vi "main.vi"() -> ()   [LabVIEW 2025]
uses:
  <vilib>/Utility/file.llb/Write Delimited Spreadsheet (DBL).vi
panel:
  out "output array":dbl[][](array[numeric])
  in  "Scrivi su File":bool
  out "Outlet":dbl
  out "Secondary":dbl
  out "Primary":dbl
  out "Waveform Graph":dynamicdata(graph)
  in  "Stop Button":bool
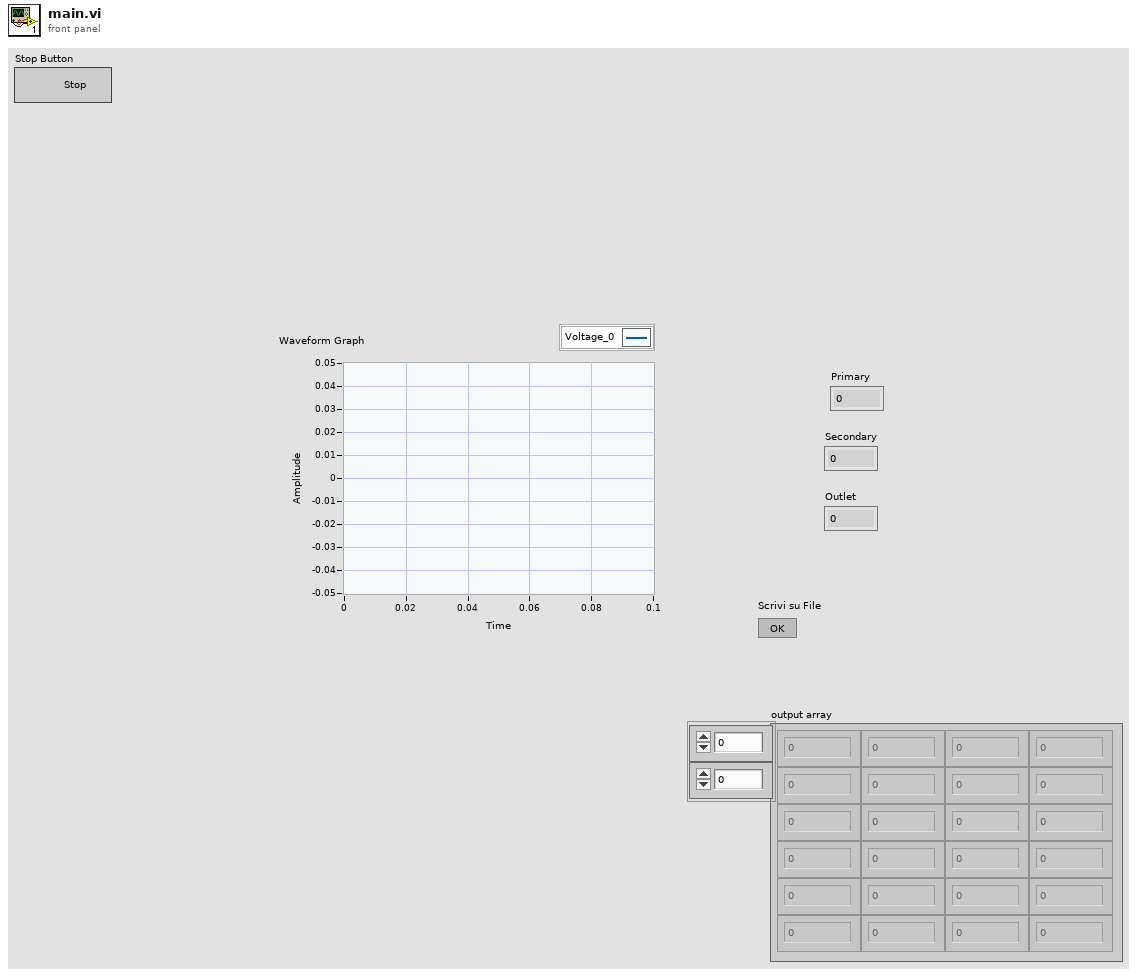
[diagram p1: front panel]
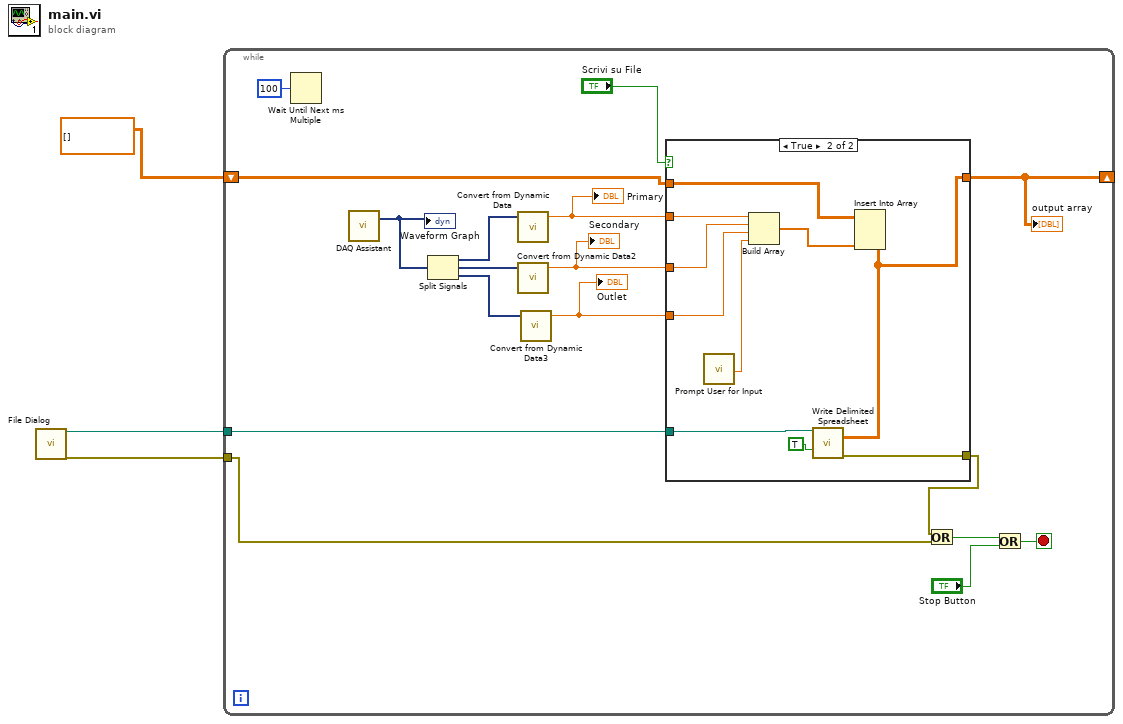
[diagram p0: block diagram]
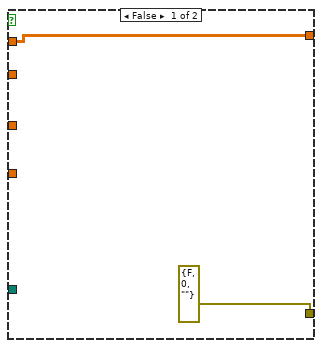
[diagram p2: hidden frame]
diagram:
  n1 = call "File Dialog"() -> ("selected path"=w3:path, "error out"=w2:errorcluster)  [unwired: 12 in, 2 out]
  n2 = while {
    tunnel: w3 -> [w9]
    tunnel: w2 -> [w7]
    shift-right: [w4] -> _
    shift-left: dbl[][] [] ("array") -> [w5]
    stop <- w14 stop-if-true
    n3 = Wait Until Next ms Multiple(millisecond multiple=u32 100) -> ()  [unwired: 1 out]
    n4 = call "DAQ Assistant"() -> ("data"=w16:dynamicdata)  [unwired: 17 in, 2 out]
    "Waveform Graph" <- w16
    n5 = Split Signals(w16) -> (w19:dynamicdata, w18:dynamicdata, w17:dynamicdata)  [unwired: 3 in]
    n6 = call "Convert from Dynamic Data"("Dynamic Data Type"=w19) -> ("Scalar"=w12:dbl)  [unwired: 3 in]
    "Primary" <- w12
    n7 = call "Convert from Dynamic Data2"("Dynamic Data Type"=w18) -> ("Scalar"=w11:dbl)  [unwired: 3 in]
    "Secondary" <- w11
    n8 = call "Convert from Dynamic Data3"("Dynamic Data Type"=w17) -> ("Scalar"=w10:dbl)  [unwired: 3 in]
    "Outlet" <- w10
    n9 = case shown="True" "Scrivi su File" {
      tunnel: w12 -> [_ w32]
      tunnel: w11 -> [_ w31]
      tunnel: w10 -> [_ w30]
      tunnel: w9 -> [_ w29]
      tunnel: [errorcluster {"status"=FALSE, "code"=0, "source"=""} ("error out") w28] -> w6
      tunnel: w5 -> [w21 w24]
      tunnel: [w21 w23] -> w4
      frame False {
      }
      frame True {
        n10 = call "Prompt User for Input"() -> ("Current"=w25:dbl)  [unwired: 17 in, 2 out]
        n11 = Build Array(w32, w31, w30, w25) -> (w27:dbl[])
        n12 = Insert Into Array(array=w24, new element=w27) -> (w23:dbl[][])  [unwired: 2 in]
        n13 = call-poly <vilib>:"Write Delimited Spreadsheet.vi"("file path (dialog if empty)"=w29, "2D data"=w23, "append to file? (new file:F)"=TRUE) -> ("error out"=w28:errorcluster)  [unwired: 11 in, 1 out]
      }
    }
    "output array" <- w4
    n14 = Or(x=w6, y=w7) -> (x .or. y?=w8:bool)
    n15 = Or(x=w8, y="Stop Button") -> (x .or. y?=w14:bool)
  }
